vi "Halverson_EMP_VStep.vi"(0 "tolerance":dbl=1e-13, 1 "Время, с":dbl=30.0, 2 "Parameter":dbl[](array[numeric])=[1.4, 1.4, 1.4], 3 "Hmax":dbl=1.0, 4 "Шаг h, с":dbl=0.01, 5 "Initial Conditions":dbl[](array[numeric])=[1.0, 0.0, 1.0], 9 "n":i32[](array[numeric])=[1, 2, 3, 4, 18, 24, 36, 24, 27, 30, 33], 10 "Ext.Type":u16(ring) items=["FNode", "MathScript", "ECD8 Arrays", "ECD8 Fnode", "ECD8 FnodeDiv", "FNode123"], 11 "k":i32=4, 12 "Multiplier":i32=4, 14 "Hmin":dbl=0.001) -> (6 "Real Error":dbl[][](graph), 15 "Output Signal":dbl[][](array[numeric]))   [LabVIEW 2016]
uses:
  <vilib>/Analysis/_algsub.llb/Real Vector Norm.vi
  <vilib>/Analysis/NI_AALPro.lvlib
panel:
  out "last value ECD1":dbl[](array[numeric])=[nan, nan, nan] format="%#_16f"
  out "Rejected Steps":i32=290950
  out "Rejected steps":i32[](graph)
  out "last value reference":dbl[](array[numeric])=[0.09918347436404504, 0.09918347436404504, 0.09918347436404504] format="%#_16f"
  out "Final time":dbl=30.001184688431483
  out "Elapsed time":dbl=5.790147253512259
  out "Number of steps":i32=29256
  out "Solution":cluster{dbl[], dbl[]}[](graph)
  out "Step Variation":dbl[](graph)
  out "Error estimation":dbl[](graph)
  in  "Error Analysis":u16(ring)=4 items=["Max", "Max_Norm", "Norm", "Last Value", "Last Constant"]
  out "Error Estimation":dbl=nan
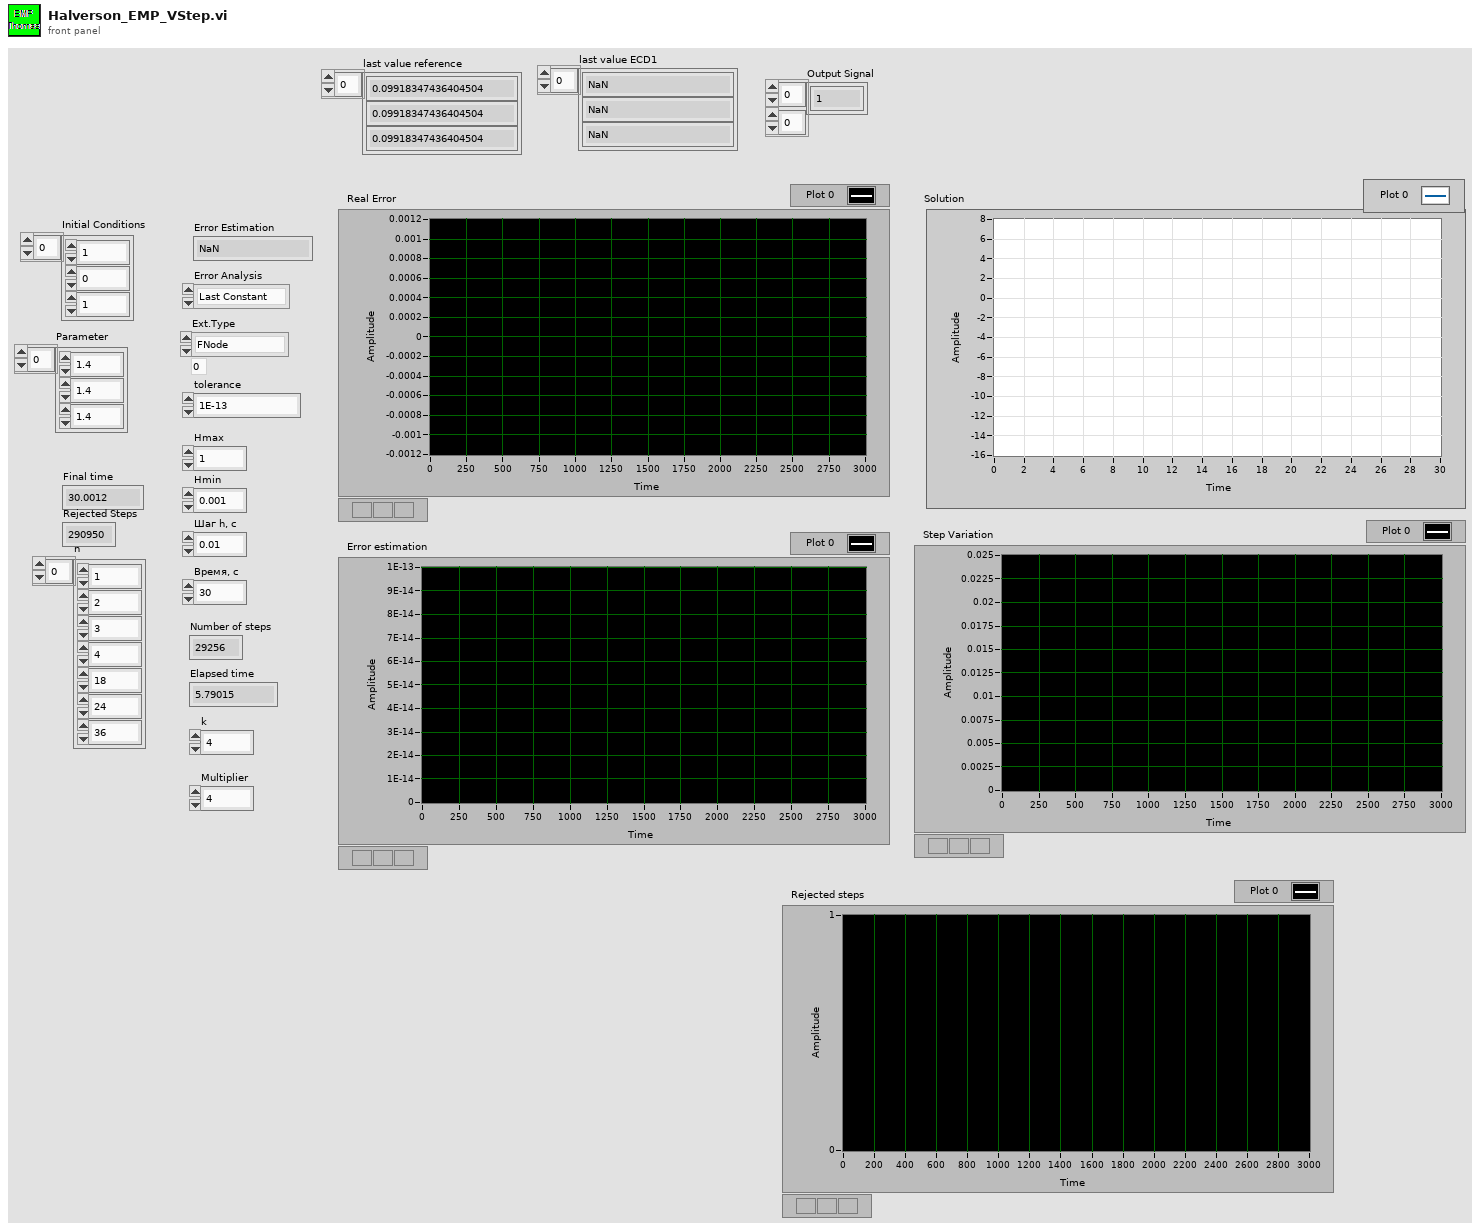
[diagram p1: front panel]
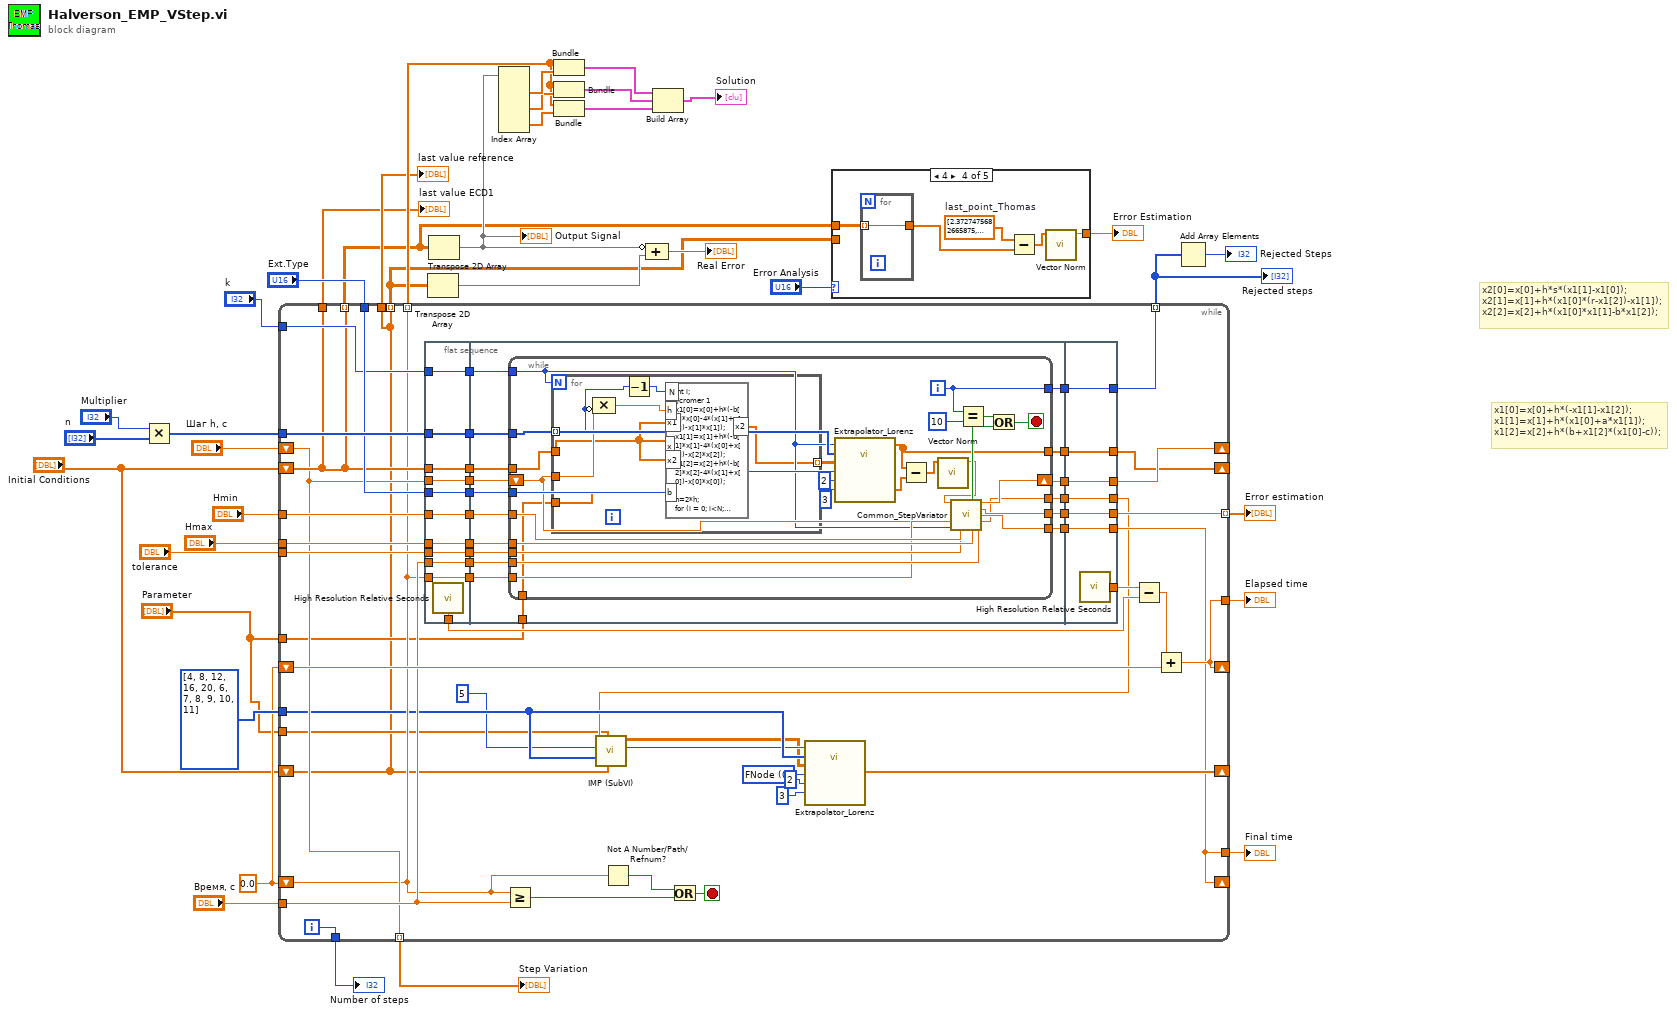
[diagram p0: block diagram]
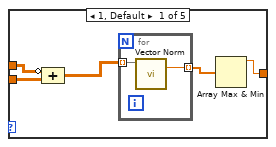
[diagram p2: hidden frame]
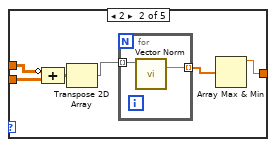
[diagram p3: hidden frame]
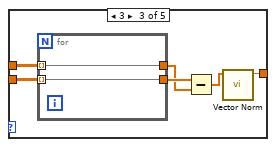
[diagram p4: hidden frame]
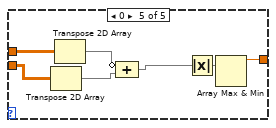
[diagram p5: hidden frame]
diagram:
  w19 = 0.0
  # "x2[0]=x[0]+h*s*(x1[1]-x1[0]);\nx2[1]=x[1]+h*(x1[0]*(r-x1[2])-x1[1]);\nx2[2]=x[2]+h*(x1[0]*x1[1]-b*x1[2]);"
  # "x1[0]=x[0]+h*(-x1[1]-x1[2]);\nx1[1]=x[1]+h*(x1[0]+a*x1[1]);\nx1[2]=x[2]+h*(b+x1[2]*(x1[0]-c));"
  n1 = Multiply(x="Multiplier", y="n") -> (x*y=w14:i32[])
  n2 = while {
    shift-right: [w60] -> _
    shift-left: "Initial Conditions" -> [w54]
    tunnel: w14 -> [w89]
    tunnel: "k" -> [w73]
    tunnel: [w54] -> w6 mode=indexing
    tunnel: "Ext.Type" -> [w87]
    shift-right: [w88] -> _
    shift-left: "Initial Conditions" -> [w39]
    tunnel: [w39] -> w5 mode=indexing
    shift-right: [w65] -> _
    shift-left: "Шаг h, с" -> [w47]
    shift-right: [w52] -> _
    shift-left: w19 -> [w46]
    tunnel: [w47] -> w33 mode=indexing
    tunnel: "Время, с" -> [w59]
    tunnel: [w46] -> w27 mode=indexing
    tunnel: [w84] -> w22
    tunnel: "tolerance" -> [w68]
    tunnel: i32[] [4, 8, 12, 16, 20, 6, 7, 8, 9, 10, 11] ("n 2") -> [w44]
    shift-right: [w75] -> _
    shift-left: w19 -> [w76]
    tunnel: [w75] -> w18
    tunnel: "Hmin" -> [w72]
    tunnel: "Hmax" -> [w70]
    tunnel: [w52] -> w12
    tunnel: [w39] -> w11
    tunnel: [w55] -> w10 mode=indexing
    tunnel: [w62] -> w8 mode=indexing
    tunnel: [w54] -> w3
    tunnel: "Parameter" -> [w40]
    tunnel: "Parameter" -> [w45]
    i -> [w84]
    stop <- w48 stop-if-true
    w51 = u16 0 items=["FNode", "MathScript", "ECD8 Arrays", "ECD8 Fnode", "ECD8 FnodeDiv"] ("Ext.Type")
    w43 = 5 ("k")
    n3 = flat-sequence {
      tunnel: w47 -> [w96]
      tunnel: w54 -> [w97]
      tunnel: w87 -> [w98]
      tunnel: w89 -> [w99]
      tunnel: w73 -> [w100]
      tunnel: [w100] -> w83
      tunnel: [w99] -> w82
      tunnel: [w98] -> w81
      tunnel: [w97] -> w80
      tunnel: [w96] -> w79
      tunnel: [w95] -> w74
      tunnel: w72 -> [w94]
      tunnel: [w94] -> w71
      tunnel: w70 -> [w93]
      tunnel: [w93] -> w69
      tunnel: w68 -> [w92]
      tunnel: [w92] -> w67
      tunnel: w59 -> [w91]
      tunnel: [w91] -> w58
      tunnel: [w90] -> w57
      tunnel: w46 -> [w90]
      tunnel: w83 -> [w113]
      tunnel: w82 -> [w112]
      tunnel: w81 -> [w117]
      tunnel: w80 -> [w111]
      tunnel: w79 -> [w110]
      tunnel: w71 -> [w116]
      tunnel: w69 -> [w115]
      tunnel: w67 -> [w114]
      tunnel: [w109] -> w66
      tunnel: [w108] -> w64
      tunnel: [w107] -> w63
      tunnel: [w106] -> w61
      tunnel: w58 -> [w105]
      tunnel: w57 -> [w104]
      tunnel: [w103] -> w56
      tunnel: [w102] -> w53
      tunnel: w45 -> [w101]
      tunnel: [w157] -> w78
      tunnel: w66 -> [w156]
      tunnel: [w156] -> w65
      tunnel: w64 -> [w155]
      tunnel: [w155] -> w42
      tunnel: w63 -> [w154]
      tunnel: [w154] -> w62
      tunnel: w61 -> [w153]
      tunnel: [w153] -> w60
      tunnel: w56 -> [w152]
      tunnel: [w152] -> w55
      tunnel: [w151] -> w52
      tunnel: w53 -> [w151]
      frame #0 {
        n4 = call <vilib>:"High Resolution Relative Seconds.vi"() -> ("relative seconds"=w95:dbl)
      }
      frame #1 {
        n5 = while {
          tunnel: w117 -> [w142]
          tunnel: w116 -> [w140]
          tunnel: w115 -> [w141]
          tunnel: w114 -> [w139]
          tunnel: w113 -> [w125]
          tunnel: w112 -> [w127]
          tunnel: w111 -> [w126]
          shift-right: [w134] -> w109
          shift-left: w110 -> [w128]
          tunnel: [w128] -> w108
          tunnel: [w133] -> w107
          tunnel: [w120] -> w106
          tunnel: w105 -> [w132]
          tunnel: w104 -> [w131]
          tunnel: [w130] -> w103
          tunnel: [w129] -> w102
          tunnel: w101 -> [w122]
          i -> [w130]
          stop <- w135 stop-if-true
          n6 = for {
            N: w125 -> [_]
            tunnel: w127 -> [w149] mode=indexing
            tunnel: w128 -> [w150]
            tunnel: w126 -> [w146]
            tunnel: [w145] -> w123 mode=indexing
            tunnel: w122 -> [w144]
            n7 = Compound Arithmetic op=MULTIPLY(w150, invert w149) -> (w147:dbl)
            n8 = Decrement(x=w149) -> (x-1=w148:i32)
            n9 = formula code="int i;\n//cromer 1\nx1[0]=x[0]+h*(-b[0]*x[0]-4*(x[1]+x[2])-x[1]*x[1]);\nx1[1]=x[1]+h*(-b[1]*x[1]-4*(x[0]+x[2])-x[2]*x[2]);\nx1[2]=x[2]+h*(-b[2]*x[2]-4*(x[1]+x[0])-x[0]*x[0]);\n\nh=2*h;\nfor (i = 0; i<N; i++)\n{\n//EEuler\nx2[0]=x[0]+h*(-b[0]*x1[0]-4*(x1[1]+x1[2])-x1[1]*x1[1]);\nx2[1]=x[1]+h*(-b[1]*x1[1]-4*(x1[0]+x1[2])-x1[2]*x1[2]);\nx2[2]=x[2]+h*(-b[2]*x1[2]-4*(x1[1]+x1[0])-x1[0]*x1[0]);\n\nx[0]=x1[0];\nx[1]=x1[1];\nx[2]=x1[2];\nx1[0]=x2[0];\nx1[1]=x2[1];\nx1[2]=x2[2];\n};"("x"=w146, "x1"=w146, "h"=w147, "x2"=w146, "N"=w148, "b"=w144) -> ("x2"=w145:dbl[])
          }
          n10 = call "Extrapolator_Lorenz.vi"("Порядок экстраполятора"=2 ("input variable"), "Dimension"=3 ("input variable"), "Ext.Type"=w142, "Х - нач. условия"=w123, "n"=w127, "k"=w125) -> ("TPrev"=w119:dbl[], "Tout"=w120:dbl[])  [unwired: 4 in]
          n11 = Subtract(x=w120, y=w119) -> (x-y=w121:dbl[])
          n12 = call-poly <vilib>:"Vector Norm.vi"("Input Vector"=w121) -> ("norm"=w118:dbl)  [unwired: 9 in, 1 out]
          n13 = call "Common_StepVariator.vi"("err"=w118, "tolerance"=w139, "Hmax"=w141, "Шаг h, с"=w128, "Current time"=w131, "k"=w125, "Hmin"=w140, "tmax"=w132) -> ("Hnew"=w134:dbl, "error estimation"=w133:dbl, "New time"=w129:dbl, "stop"=w136:bool)  [unwired: 4 in]
          n14 = Equal?(x=w130, y=10) -> (x = y?=w137:bool)
          n15 = Or(x=w137, y=w136) -> (x .or. y?=w135:bool)
        }
      }
      frame #2 {
        n16 = call <vilib>:"High Resolution Relative Seconds.vi"() -> ("relative seconds"=w157:dbl)
      }
    }
    n17 = Greater Or Equal?(x=w46, y=w59) -> (x >= y?=w49:bool)
    n18 = call "IMP (SubVI).vi"("Initial Conditions in"=w39, "b"=w40, "n in"=w44, "Numeric"=w43, "Шаг h, с"=w42) -> ("Initial Conditions out"=w41:dbl[][])  [unwired: 6 in]
    n19 = Not A Number/Path/Refnum?(number/path/refnum=w46) -> (NaN/Path/Refnum?=w50:bool)
    n20 = Or(x=w50, y=w49) -> (x .or. y?=w48:bool)
    n21 = call "Extrapolator_Lorenz.vi"("Порядок экстраполятора"=2, "Dimension"=3, "Ext.Type"=w51, "Х - нач. условия"=w41, "n"=w44, "k"=w43) -> ("Tout"=w88:dbl[])  [unwired: 4 in, 1 out]
    n22 = Subtract(x=w78, y=w74) -> (x-y=w77:dbl)
    n23 = Add(x=w77, y=w76) -> (x+y=w75:dbl)
  }
  "Error estimation" <- w8
  "Step Variation" <- w33
  "Number of steps" <- w22
  "Elapsed time" <- w18
  "Final time" <- w12
  "last value reference" <- w11
  "Rejected steps" <- w10
  "last value ECD1" <- w3
  n24 = Transpose 2D Array(2D array=w5) -> (transposed array=w34:dbl[][])
  n25 = Transpose 2D Array(2D array=w6) -> (transposed array=w31:dbl[][])
  "Output Signal" <- w31
  n26 = Index Array(array=w31) -> (element #1=w30:dbl[], element #2=w29:dbl[], element #3=w28:dbl[])  [unwired: 6 in]
  n27 = Bundle(w27, w30) -> (w26:cluster{dbl[], dbl[]})  [unwired: 1 in]
  n28 = Bundle(w27, w29) -> (w25:cluster{dbl[], dbl[]})  [unwired: 1 in]
  n29 = Bundle(w27, w28) -> (w24:cluster{dbl[], dbl[]})  [unwired: 1 in]
  n30 = Compound Arithmetic op=ADD(invert w31, w34) -> (→"Real Error":dbl[][])
  n31 = Build Array(w26, w25, w24) -> (→"Solution":cluster{dbl[], dbl[]}[])
  n32 = case shown="4" "Error Analysis" {
    tunnel: w5 -> [w159 w167 w176 _ w187]
    tunnel: [w161 w169 w178 w185 w192] -> w4
    tunnel: w6 -> [w160 w168 w177 w184 w188]
    frame 1, Default {
      n33 = Compound Arithmetic op=ADD(invert w160, w159) -> (w158:dbl[][])
      n34 = for {
        tunnel: [w164] -> w162 mode=indexing
        tunnel: w158 -> [w163] mode=indexing
        n35 = call-poly <vilib>:"Vector Norm.vi"("Input Vector"=w163) -> ("norm"=w164:dbl)  [unwired: 9 in, 1 out]
      }
      n36 = Array Max & Min(array=w162) -> (max value=w161:dbl)  [unwired: 3 out]
    }
    frame 2 {
      n37 = Compound Arithmetic op=ADD(invert w168, w167) -> (w166:dbl[][])
      n38 = Transpose 2D Array(2D array=w166) -> (transposed array=w165:dbl[][])
      n39 = for {
        tunnel: [w172] -> w170 mode=indexing
        tunnel: w165 -> [w171] mode=indexing
        n40 = call-poly <vilib>:"Vector Norm.vi"("Input Vector"=w171) -> ("norm"=w172:dbl)  [unwired: 9 in, 1 out]
      }
      n41 = Array Max & Min(array=w170) -> (max value=w169:dbl)  [unwired: 3 out]
    }
    frame 3 {
      n42 = for {
        tunnel: w177 -> [w180] mode=indexing
        tunnel: [w180] -> w174
        tunnel: w176 -> [w179] mode=indexing
        tunnel: [w179] -> w175
      }
      n43 = Subtract(x=w175, y=w174) -> (x-y=w173:dbl[])
      n44 = call-poly <vilib>:"Vector Norm.vi"("Input Vector"=w173) -> ("norm"=w178:dbl)  [unwired: 9 in, 1 out]
    }
    frame 4 {
      w181 = dbl[] [2.3727475682665875, 0.23609824454436878, 0.4447912442126299]  # last_point_Thomas
      n45 = for {
        tunnel: w184 -> [w186] mode=indexing
        tunnel: [w186] -> w183
      }
      n46 = Subtract(x=w181, y=w183) -> (x-y=w182:dbl[])
      n47 = call-poly <vilib>:"Vector Norm.vi"("Input Vector"=w182) -> ("norm"=w185:dbl)  [unwired: 9 in, 1 out]
    }
    frame 0 {
      n48 = Transpose 2D Array(2D array=w187) -> (transposed array=w190:dbl[][])
      n49 = Transpose 2D Array(2D array=w188) -> (transposed array=w191:dbl[][])
      n50 = Compound Arithmetic op=ADD(invert w191, w190) -> (w189:dbl[][])
      n51 = Absolute Value(x=w189) -> (abs(x)=w193:dbl[][])
      n52 = Array Max & Min(array=w193) -> (max value=w192:dbl)  [unwired: 3 out]
    }
  }
  "Error Estimation" <- w4
  n53 = Add Array Elements(numeric array=w10) -> (sum=→"Rejected Steps":i32)
